vi "GDSError_ClearError.vi"(2 "code":i32=5000, 3 "codes":i32[](array[numeric]), 5 "error in (no error)":errorcluster, 7 "Message popup":string, 9 "Message popups":string[](array[string])) -> (16 "Cleared?":bool, 19 "error out":errorcluster)   [LabVIEW 2014]
doc: "Use this VI to ignore errors with a certain code."
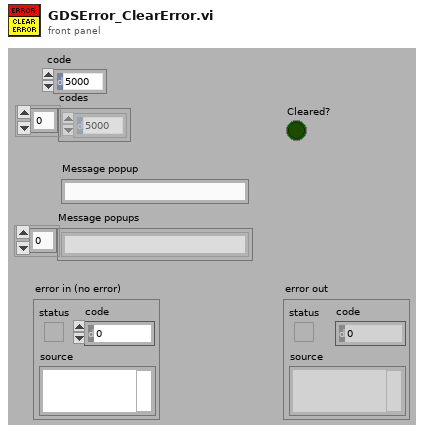
[diagram p1: front panel]
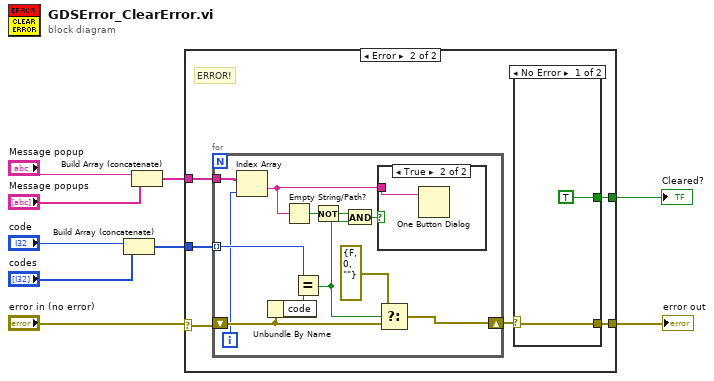
[diagram p0: block diagram]
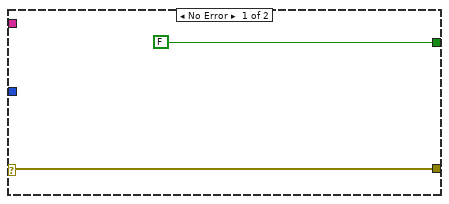
[diagram p2: hidden frame]
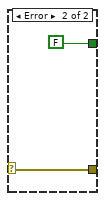
[diagram p3: hidden frame]
diagram:
  n1 = Build Array (concatenate)("code", "codes") -> (w4:i32[])
  n2 = Build Array (concatenate)("Message popup", "Message popups") -> (w1:string[])
  n3 = case shown="Error" "error in (no error)" {
    selector: "error in (no error)" -> [w10 w17]
    tunnel: [w10 w13] -> w9
    tunnel: [FALSE w14] -> w8
    tunnel: w4 -> [_ w16]
    tunnel: w1 -> [_ w12]
    frame No Error {
    }
    frame Error {
      # "ERROR!"
      n4 = for {
        shift-right: [w30] -> w15
        shift-left: w17 -> [w31]
        tunnel: w16 -> [w29] mode=indexing
        tunnel: w12 -> [w28]
        i -> [w25]
        n5 = Index Array(array=w28, index=w25) -> (element=w24:string)
        n6 = Unbundle By Name(w31) -> ("code"=w33:i32)
        n7 = Empty String/Path?(string/path=w24) -> (empty?=w23:bool)
        n8 = Equal?(x=w29, y=w33) -> (x = y?=w27:bool)
        n9 = Not(x=w23) -> (.not. x?=w22:bool)
        n10 = And(x=w22, y=w27) -> (x .and. y?=w26:bool)
        n11 = case shown="True" w26 {
          tunnel: w24 -> [_ w34]
          frame False {
          }
          frame True {
            n12 = One Button Dialog(message=w34) -> ()  [unwired: 1 in, 1 out]
          }
        }
        n13 = Select(t=errorcluster {"status"=FALSE, "code"=0, "source"=""}, s=w27, f=w31) -> (s? t:f=w30:errorcluster)
      }
      n14 = case shown="No Error" w15 {
        selector: w15 -> [w18 w20]
        tunnel: [TRUE FALSE] -> w14
        tunnel: [w18 w20] -> w13
        frame No Error {
        }
        frame Error {
        }
      }
    }
  }
  "error out" <- w9
  "Cleared?" <- w8
